vi "visuallyInspectPositionListResults2.vi"() -> ()   [LabVIEW 2016]
uses:
  <vilib>/Utility/file.llb/Write Delimited Spreadsheet (DBL).vi
  <vilib>/regexp/Match Regular Expression.xnode
  <vilib>/vision/driver/NI_Vision_Acquisition_Software.lvlib
  <vilib>/vision/NI_Vision_Development_Module.lvlib
panel:
  out "Array":dbl[][](array[numeric])=[[169.71, 122.239, 18.9126], [169.219, 25.0888, 17.9835], [73.8248, 25.6014, 13.716], [74.3048, 122.763, 15.0633], [169.71, 122.239, 18.9126], [169.219, 25.0888, 17.9835], [73.8248, 25.6014, 13.716], [74.3048, 122.763, 15.0633], [169.71, 122.239, 18.9126], [169.219, 25.0888, 17.9835], [73.8248, 25.6014, 13.716], [74.3048, 122.763, 15.0633], [169.71, 122.239, 18.9126], [169.219, 25.0888, 17.9835], [73.8248, 25.6014, 13.716], [74.3048, 122.763, 15.0633], [169.71, 122.239, 18.9126], [169.219, 25.0888, 17.9835], [73.8248, 25.6014, 13.716], [74.3048, 122.763, 15.0633], [169.71, 122.239, 18.9126], [169.219, 25.0888, 17.9835], [73.8248, 25.6014, 13.716], [74.3048, 122.763, 15.0633], [169.71, 122.239, 18.9126], [169.219, 25.0888, 17.9835], [73.8248, 25.6014, 13.716], [74.3048, 122.763, 15.0633], [169.71, 122.239, 18.9126], [169.219, 25.0888, 17.9835], [73.8248, 25.6014, 13.716], [74.3048, 122.763, 15.0633], [169.71, 122.239, 18.9126], [169.219, 25.0888, 17.9835], [73.8248, 25.6014, 13.716], [74.3048, 122.763, 15.0633], [169.71, 122.239, 18.9126], [169.219, 25.0888, 17.9835], [73.8248, 25.6014, 13.716], [74.3048, 122.763, 15.0633]]
  in  "Tab Control":T1(tab)
  in  "Path to save collected images":path=path "C:/Users/Aerotech/Downloads/Test"
  in  "List of Interesting Locations":path=path "C:/Users/Aerotech/Downloads/Test/coords.csv"
  out "Pixel Y":dbl=1374.0
  out "Pixel X":dbl=1920.0
  in  "Nloops":i32=1
  in  "Ncaptures":i32=1
  in  "File delimiter":string=","
  out "Number of Images":i32=160
  in  "Camera gain":dbl(slide)=3.6197718631178706 scale=0.0..16.0
  out "Thermometer [C]":dbl(slide)=nan scale=0.0..50.0
  in  "Coaxial light":bool
  in  "Spotlights":bool
  out "XYZ Stage Current Position":T2={"X [-750, 750 mm]"=74.30480031245196, "Y [-150, 30 mm]"=122.76299520213085, "Z [-50, 50 mm]"=15.0633357184}
  out "Finished!":bool
  in  "Home?":bool
  in  "Focusing test range [mm]":dbl=0.8
  in  "Stepsize [um]":dbl=200.0
  in  "Scan height?":bool
  in  "Axes Speeds [mm/s]":T3={"X Speed"=30.0, "Y Speed"=30.0, "Z Speed"=15.0}
  in  "Milliseconds to Wait":u32=5000
  in  "Camera Name":refnum<k21>="cam0" caption="IMAQdx Session"
  in  "Object Location [mm]":T4={"Go to X"=74.3048, "Go to Y"=122.763, "Go to Z"=15.0633}
  out "Moving":bool
  in  "Set of Coordinates to Process":dbl[][](array[numeric])=[[169.71, 122.239, 18.9126], [169.71, 122.239, 18.9126], [169.71, 122.239, 18.9126], [169.71, 122.239, 18.9126], [169.219, 25.0888, 17.9835], [169.219, 25.0888, 17.9835], [169.219, 25.0888, 17.9835], [169.219, 25.0888, 17.9835], [73.8248, 25.6014, 13.716], [73.8248, 25.6014, 13.716], [73.8248, 25.6014, 13.716], [73.8248, 25.6014, 13.716], [74.3048, 122.763, 15.0633], [74.3048, 122.763, 15.0633], [74.3048, 122.763, 15.0633], [74.3048, 122.763, 15.0633], [169.71, 122.239, 18.9126], [169.71, 122.239, 18.9126], [169.71, 122.239, 18.9126], [169.71, 122.239, 18.9126], [169.219, 25.0888, 17.9835], [169.219, 25.0888, 17.9835], [169.219, 25.0888, 17.9835], [169.219, 25.0888, 17.9835], [73.8248, 25.6014, 13.716], [73.8248, 25.6014, 13.716], [73.8248, 25.6014, 13.716], [73.8248, 25.6014, 13.716], [74.3048, 122.763, 15.0633], [74.3048, 122.763, 15.0633], [74.3048, 122.763, 15.0633], [74.3048, 122.763, 15.0633], [169.71, 122.239, 18.9126], [169.71, 122.239, 18.9126], [169.71, 122.239, 18.9126], [169.71, 122.239, 18.9126], [169.219, 25.0888, 17.9835], [169.219, 25.0888, 17.9835], [169.219, 25.0888, 17.9835], [169.219, 25.0888, 17.9835], [73.8248, 25.6014, 13.716], [73.8248, 25.6014, 13.716], [73.8248, 25.6014, 13.716], [73.8248, 25.6014, 13.716], [74.3048, 122.763, 15.0633], [74.3048, 122.763, 15.0633], [74.3048, 122.763, 15.0633], [74.3048, 122.763, 15.0633], [169.71, 122.239, 18.9126], [169.71, 122.239, 18.9126], [169.71, 122.239, 18.9126], [169.71, 122.239, 18.9126], [169.219, 25.0888, 17.9835], [169.219, 25.0888, 17.9835], [169.219, 25.0888, 17.9835], [169.219, 25.0888, 17.9835], [73.8248, 25.6014, 13.716], [73.8248, 25.6014, 13.716], [73.8248, 25.6014, 13.716], [73.8248, 25.6014, 13.716], [74.3048, 122.763, 15.0633], [74.3048, 122.763, 15.0633], [74.3048, 122.763, 15.0633], [74.3048, 122.763, 15.0633], [169.71, 122.239, 18.9126], [169.71, 122.239, 18.9126], [169.71, 122.239, 18.9126], [169.71, 122.239, 18.9126], [169.219, 25.0888, 17.9835], [169.219, 25.0888, 17.9835], [169.219, 25.0888, 17.9835], [169.219, 25.0888, 17.9835], [73.8248, 25.6014, 13.716], [73.8248, 25.6014, 13.716], [73.8248, 25.6014, 13.716], [73.8248, 25.6014, 13.716], [74.3048, 122.763, 15.0633], [74.3048, 122.763, 15.0633], [74.3048, 122.763, 15.0633], [74.3048, 122.763, 15.0633], [169.71, 122.239, 18.9126], [169.71, 122.239, 18.9126], [169.71, 122.239, 18.9126], [169.71, 122.239, 18.9126], [169.219, 25.0888, 17.9835], [169.219, 25.0888, 17.9835], [169.219, 25.0888, 17.9835], [169.219, 25.0888, 17.9835], [73.8248, 25.6014, 13.716], [73.8248, 25.6014, 13.716], [73.8248, 25.6014, 13.716], [73.8248, 25.6014, 13.716], [74.3048, 122.763, 15.0633], [74.3048, 122.763, 15.0633], [74.3048, 122.763, 15.0633], [74.3048, 122.763, 15.0633], [169.71, 122.239, 18.9126], [169.71, 122.239, 18.9126], [169.71, 122.239, 18.9126], [169.71, 122.239, 18.9126], [169.219, 25.0888, 17.9835], [169.219, 25.0888, 17.9835], [169.219, 25.0888, 17.9835], [169.219, 25.0888, 17.9835], [73.8248, 25.6014, 13.716], [73.8248, 25.6014, 13.716], [73.8248, 25.6014, 13.716], [73.8248, 25.6014, 13.716], [74.3048, 122.763, 15.0633], [74.3048, 122.763, 15.0633], [74.3048, 122.763, 15.0633], [74.3048, 122.763, 15.0633], [169.71, 122.239, 18.9126], [169.71, 122.239, 18.9126], [169.71, 122.239, 18.9126], [169.71, 122.239, 18.9126], [169.219, 25.0888, 17.9835], [169.219, 25.0888, 17.9835], [169.219, 25.0888, 17.9835], [169.219, 25.0888, 17.9835], [73.8248, 25.6014, 13.716], [73.8248, 25.6014, 13.716], [73.8248, 25.6014, 13.716], [73.8248, 25.6014, 13.716], [74.3048, 122.763, 15.0633], [74.3048, 122.763, 15.0633], [74.3048, 122.763, 15.0633], [74.3048, 122.763, 15.0633], [169.71, 122.239, 18.9126], [169.71, 122.239, 18.9126], [169.71, 122.239, 18.9126], [169.71, 122.239, 18.9126], [169.219, 25.0888, 17.9835], [169.219, 25.0888, 17.9835], [169.219, 25.0888, 17.9835], [169.219, 25.0888, 17.9835], [73.8248, 25.6014, 13.716], [73.8248, 25.6014, 13.716], [73.8248, 25.6014, 13.716], [73.8248, 25.6014, 13.716], [74.3048, 122.763, 15.0633], [74.3048, 122.763, 15.0633], [74.3048, 122.763, 15.0633], [74.3048, 122.763, 15.0633], [169.71, 122.239, 18.9126], [169.71, 122.239, 18.9126], [169.71, 122.239, 18.9126], [169.71, 122.239, 18.9126], [169.219, 25.0888, 17.9835], [169.219, 25.0888, 17.9835], [169.219, 25.0888, 17.9835], [169.219, 25.0888, 17.9835], [73.8248, 25.6014, 13.716], [73.8248, 25.6014, 13.716], [73.8248, 25.6014, 13.716], [73.8248, 25.6014, 13.716], [74.3048, 122.763, 15.0633], [74.3048, 122.763, 15.0633], [74.3048, 122.763, 15.0633], [74.3048, 122.763, 15.0633]]
  in  "Settings":T5={"Algorithm"=2, "Number of Matches Requested"=1, "Minimum Match Score"=800.0, "SubPixel Accuracy"=TRUE, "Rotation Angle Ranges"=[], "Show Search Area"=FALSE, "Show Result"=TRUE} {"Rotation Angle Ranges"."End" format="%.1f"; "Rotation Angle Ranges"."Start" format="%.1f"; "Minimum Match Score" min=0 max=1000 format="%.2f"; "Number of Matches Requested" min=1; "Algorithm" items=["All", "Low Discrepancy Sampling", "Grayscale Value Pyramid", "Gradients Pyramid"]}
  out "Most recently collected image":T6(plugin-control)
  out "Image #":i32=159
  in  "error in (no error)":errorcluster
  out "Error report":errorcluster
  out "VISA error out":errorcluster={"status"=TRUE, "code"=5002, "source"="Init.vi.  Unable to establish connection with Arduino.  Please ensure that you have selected the correct COM port and that you have flashed the Arduino with the correct firmware."}
  # "This VI can take pictures save the coordinates \nIt can also do the pattern matching at fly\nDifferent pattern could be matched but the template must be in the correct folder\nThe matched coordinates are in pixel which is to be later connverted into mm"
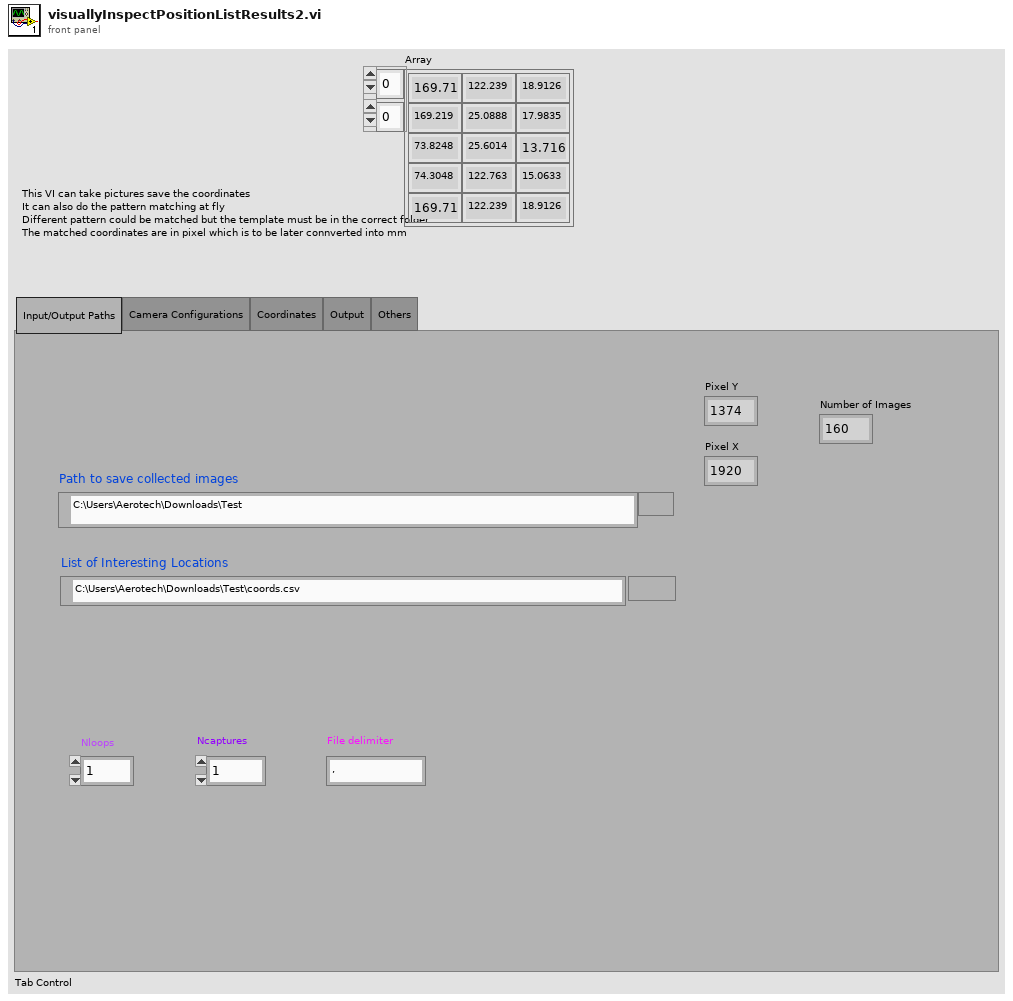
[diagram p1: front panel]
types:
  T1 = enum32{"Input/Output Paths", "Camera Configurations", "Coordinates", "Output", "Others"}
  T2 = cluster{"X [-750, 750 mm]":dbl, "Y [-150, 30 mm]":dbl, "Z [-50, 50 mm]":dbl}
  T3 = cluster{"X Speed":dbl, "Y Speed":dbl, "Z Speed":dbl}
  T4 = cluster{"Go to X":dbl, "Go to Y":dbl, "Go to Z":dbl}
  T5 = cluster{"Algorithm":i32, "Number of Matches Requested":i32, "Minimum Match Score":sgl, "SubPixel Accuracy":bool, "Rotation Angle Ranges":cluster{"Start":sgl, "End":sgl}[], "Show Search Area":bool, "Show Result":bool}
  T6 = typedef "IMAQ Image.ctl" = refnum<image>
  T7 = cluster{"Loaded array[0]":dbl, "Loaded array[1]":dbl, "Loaded array[2]":dbl, "Loaded array[3]":dbl, "Loaded array[4]":dbl, "Loaded array[5]":dbl, "Loaded array[6]":dbl, "Loaded array[7]":dbl, "Loaded array[8]":dbl}
  T8 = typedef "LabVIEW Interface for Arduino.lvlib/Arduino Resource.ctl" = cluster{"VISA resource":refnum<visa-resource-name>, "Board Type":T9, "Connection Type":enum8{"USB / Serial"}, "Bytes Per Packet (15)":u8}
  T9 = typedef "LabVIEW Interface for Arduino.lvlib/Board Type.ctl" = enum16{"Uno", "Dimuelanove w/Atmega 328", "Mega 2560"}
  T10 = typedef "ArduinoLT-ConfigurationControl.ctl" = cluster{"Lights: Digital I/O Pins":cluster{"Coaxial":u8, "Spotlights":u8}, "Thermistor Settings":cluster{"Analogue Readout Pin":u8, "Vcc Reference Pin":u8, "Paired Resistance (10K Ohms)":dbl, "Units (C)":enum16{"Celsius", "Fahrenheit", "Kelvin"}}}
  T11 = typedef "IMAQdx.ctl" = refnum<k21>
  T12 = cluster{"Set of Coordinates to Process[0]":dbl, "Set of Coordinates to Process[1]":dbl, "Set of Coordinates to Process[2]":dbl}
  T13 = typedef "Image Type" = u32
  T14 = cluster{"Final X":dbl, "Final Y":dbl, "Final Z":dbl}
  T15 = cluster{"Position":cluster{"x":sgl, "y":sgl}, "Angle":sgl, "Scale":sgl, "Score":sgl, "Bounding Box":cluster{"x":sgl, "y":sgl}[]}[]
  T16 = cluster{"Matches (pixel)[0]":cluster{"Position":cluster{"x":sgl, "y":sgl}, "Angle":sgl, "Scale":sgl, "Score":sgl, "Bounding Box":cluster{"x":sgl, "y":sgl}[]}, "Matches (pixel)[1]":cluster{"Position":cluster{"x":sgl, "y":sgl}, "Angle":sgl, "Scale":sgl, "Score":sgl, "Bounding Box":cluster{"x":sgl, "y":sgl}[]}, "Matches (pixel)[2]":cluster{"Position":cluster{"x":sgl, "y":sgl}, "Angle":sgl, "Scale":sgl, "Score":sgl, "Bounding Box":cluster{"x":sgl, "y":sgl}[]}, "Matches (pixel)[3]":cluster{"Position":cluster{"x":sgl, "y":sgl}, "Angle":sgl, "Scale":sgl, "Score":sgl, "Bounding Box":cluster{"x":sgl, "y":sgl}[]}, "Matches (pixel)[4]":cluster{"Position":cluster{"x":sgl, "y":sgl}, "Angle":sgl, "Scale":sgl, "Score":sgl, "Bounding Box":cluster{"x":sgl, "y":sgl}[]}, "Matches (pixel)[5]":cluster{"Position":cluster{"x":sgl, "y":sgl}, "Angle":sgl, "Scale":sgl, "Score":sgl, "Bounding Box":cluster{"x":sgl, "y":sgl}[]}, "Matches (pixel)[6]":cluster{"Position":cluster{"x":sgl, "y":sgl}, "Angle":sgl, "Scale":sgl, "Score":sgl, "Bounding Box":cluster{"x":sgl, "y":sgl}[]}, "Matches (pixel)[7]":cluster{"Position":cluster{"x":sgl, "y":sgl}, "Angle":sgl, "Scale":sgl, "Score":sgl, "Bounding Box":cluster{"x":sgl, "y":sgl}[]}, "Matches (pixel)[8]":cluster{"Position":cluster{"x":sgl, "y":sgl}, "Angle":sgl, "Scale":sgl, "Score":sgl, "Bounding Box":cluster{"x":sgl, "y":sgl}[]}}
  T17 = cluster{"Position":cluster{"x":sgl, "y":sgl}, "Angle":sgl, "Scale":sgl, "Score":sgl, "Bounding Box":cluster{"x":sgl, "y":sgl}[]}
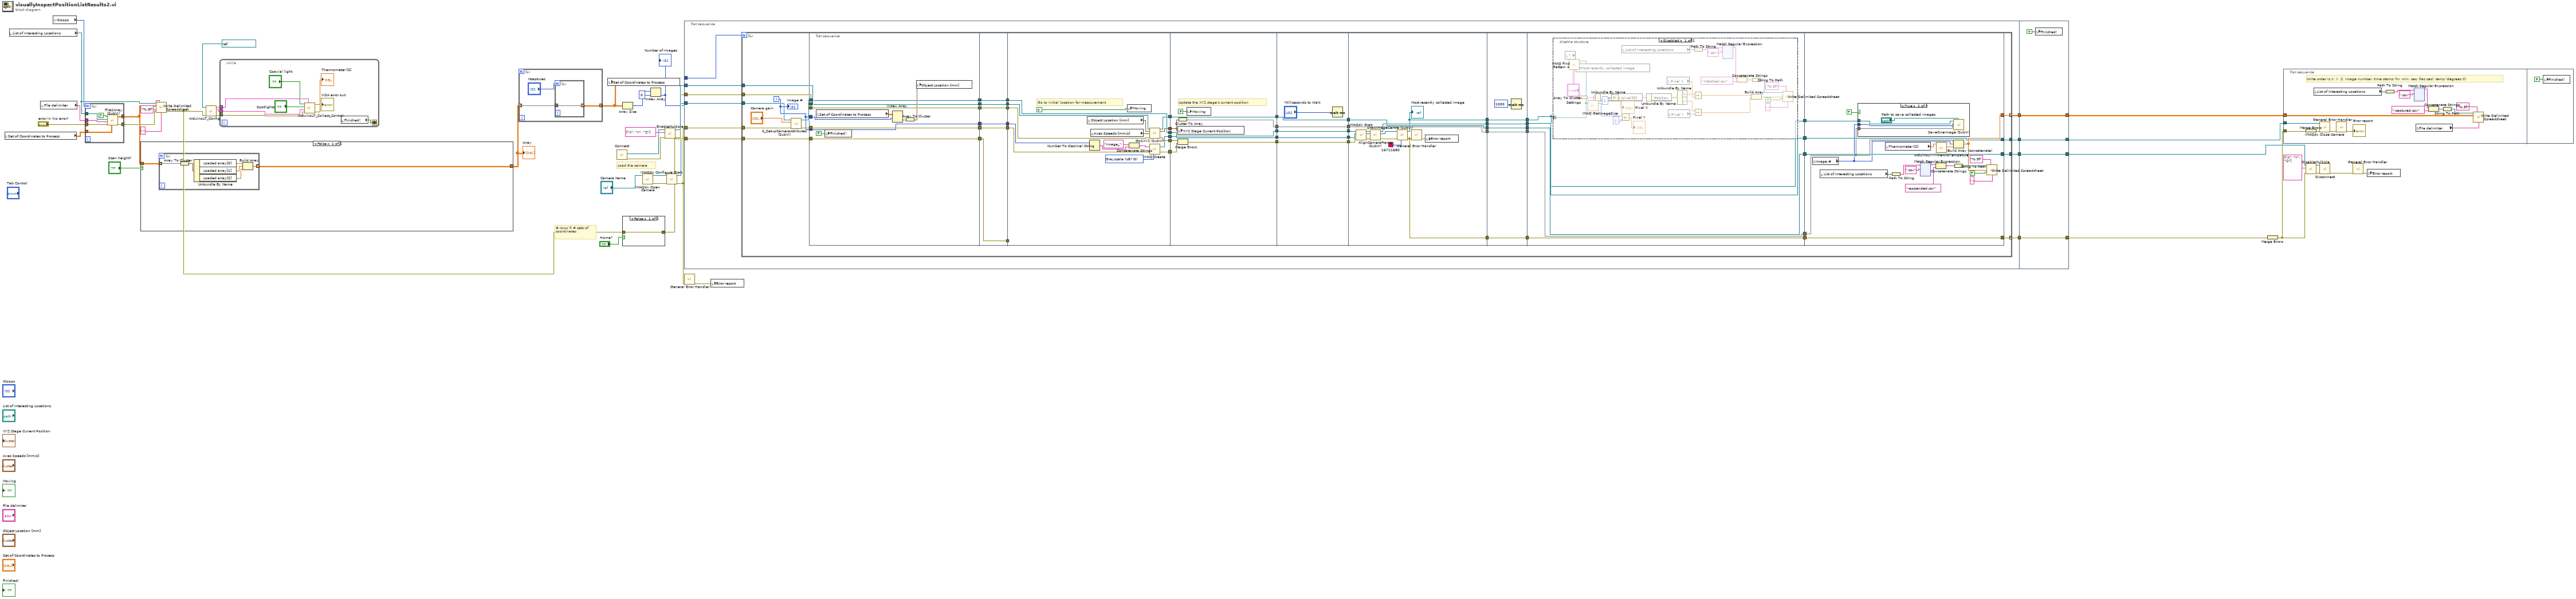
[diagram p0: block diagram]
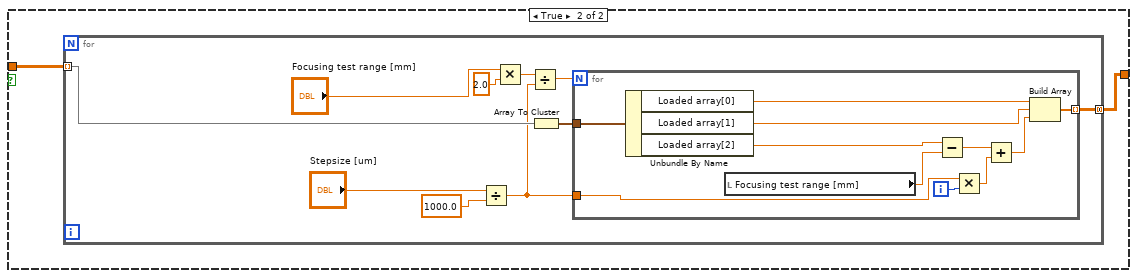
[diagram p2: hidden frame]
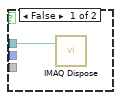
[diagram p4: hidden frame]
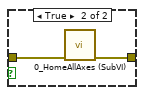
[diagram p5: hidden frame]
diagram:
  # "# rows = # sets of\ncoordinates"
  # "Load the camera"
  n1 = local read "Set of Coordinates to Process"() -> (w36:dbl[][])
  n2 = local read "List of Interesting Locations"() -> (w35:path)
  n3 = local read "File delimiter"() -> (w38:string)
  n4 = local read "Nloops"() -> (w15:i32)
  n5 = for {
    N: w15 -> [_]
    tunnel: w35 -> [w51]
    tunnel: w38 -> [w50]
    tunnel: w36 -> [w48]
    tunnel: [w54] -> w17 mode=concatenating
    tunnel: "error in (no error)" -> [w49]
    tunnel: [w53] -> w13
    n6 = call "File2Array (SubVI).vi"("Array for Processing"=w48, "error in (no error) in"=w49, "File delimiter"=w50, "Source array file"=w51, "Load array from file?"=TRUE) -> ("error in (no error) out"=w53:errorcluster, "Loaded array"=w54:dbl[][])  [unwired: 5 in]
  }
  n7 = case shown="False" "Scan height?" {
    tunnel: w17 -> [w56 w64]
    tunnel: [w55 w63] -> w16
    frame False {
      n8 = for {
        tunnel: w56 -> [w62] mode=indexing
        tunnel: [w58] -> w55 mode=indexing
        n9 = Array To Cluster(array=w62) -> (cluster=w61:T7)
        n10 = Unbundle By Name(w61) -> ("Loaded array[0]"=w60:dbl, "Loaded array[1]"=w59:dbl, "Loaded array[2]"=w57:dbl)
        n11 = Build Array(w60, w59, w57) -> (w58:dbl[])
      }
    }
    frame True {
      n12 = for {
        tunnel: w64 -> [w70] mode=indexing
        tunnel: [w68] -> w63 mode=concatenating
        n13 = Divide(x="Stepsize [um]", y=1000.0) -> (x/y=w65:dbl)
        n14 = Multiply(x="Focusing test range [mm]", y=2.0) -> (x*y=w72:dbl)
        n15 = Divide(x=w72, y=w65) -> (x/y=w73:dbl)
        n16 = Array To Cluster(array=w70) -> (cluster=w69:T7)
        n17 = for {
          N: w73 -> [_]
          tunnel: w69 -> [w85]
          tunnel: [w82] -> w68 mode=indexing
          tunnel: w65 -> [w80]
          i -> [w81]
          n18 = Unbundle By Name(w85) -> ("Loaded array[0]"=w84:dbl, "Loaded array[1]"=w83:dbl, "Loaded array[2]"=w79:dbl)
          n19 = local read "Focusing test range [mm]"() -> (w78:dbl)
          n20 = Subtract(x=w79, y=w78) -> (x-y=w77:dbl)
          n21 = Multiply(x=w80, y=w81) -> (x*y=w76:dbl)
          n22 = Add(x=w77, y=w76) -> (x+y=w75:dbl)
          n23 = Build Array(w84, w83, w75) -> (w82:dbl[])
        }
      }
    }
  }
  "Array" <- w16
  n24 = call-poly <vilib>:"Write Delimited Spreadsheet.vi"("file path (dialog if empty)"=w35, "format (%.3f)"="%.9f", "2D data"=w17, "error in (no error)"=w13, "delimiter (\\t)"="," ("delimiter (\\t)")) -> ("error out"=w9:errorcluster)  [unwired: 9 in, 1 out]
  n25 = call "ArduinoLT_Config.vi"("error in"=w9, "VISA resource"=refnum<visa-resource-name> "LightsCTRL") -> ("error out"=w5:errorcluster, "Arduino Resource"=w8:T8, "Arduino Configuration OUT"=w7:T10)  [unwired: 3 in, 1 out]
  n26 = while {
    tunnel: w8 -> [w89]
    tunnel: w7 -> [w88]
    tunnel: w5 -> [w87]
    stop <- w90 stop-if-true
    n27 = call "ArduinoLT_Collect_Control.vi"("Arduino Configuration"=w88, "error in"=w87, "Arduino Resource IN"=w89, "Spotlights"="Spotlights", "Coaxial light"="Coaxial light") -> ("error out"=→"VISA error out":errorcluster, "Thermometer [C]"=→"Thermometer [C]":dbl)  [unwired: 4 in, 1 out]
    n28 = local read "Finished!"() -> (w90:bool)
  }
  n29 = for {
    tunnel: w16 -> [w95] mode=indexing
    tunnel: [w94] -> w1 mode=concatenating
    n30 = for {
      N: "Ncaptures" -> [_]
      tunnel: w95 -> [w97]
      tunnel: [w97] -> w94 mode=indexing
    }
  }
  n31 = local write "Set of Coordinates to Process"(w1) -> ()
  n32 = call "Connect.vi"() -> ("error out"=w29:errorcluster, "controller"=w28:refnum<k24>)  [unwired: 10 in]
  n33 = Array Size(array=w1) -> (size(s)=w3:i32[])
  n34 = case shown="False" "Home?" {
    tunnel: w9 -> [w98 w100]
    tunnel: [w98 w99] -> w42
    frame False {
    }
    frame True {
      n35 = call "0_HomeAllAxes (SubVI).vi"("error in (no error)"=w100) -> ("error out"=w99:errorcluster)  [unwired: 7 in, 3 out]
    }
  }
  n36 = call <vilib>:"IMAQdx Open Camera.vi"("Session In"="Camera Name") -> ("error out"=w46:errorcluster, "Session Out"=w47:T11)  [unwired: 2 in, 7 out]
  n37 = Index Array(array=w3, index=0) -> (element=w2:i32)
  "Number of Images" <- w2
  n38 = call "EnableMultiple.vi"("error in (no error)"=w29, "axis names"=string[] ["X", "Y", "Z"], "controller in"=w28) -> ("error out"=w26:errorcluster, "controller out"=w27:refnum<k24>)  [unwired: 7 in]
  n39 = call <vilib>:"IMAQdx Configure Grab.vi"("error in"=w46, "Session In"=w47) -> ("error out"=w10:errorcluster, "Session Out"=w11:T11)  [unwired: 8 out]
  n40 = flat-sequence {
    tunnel: [w109] -> w34
    tunnel: [w103] -> w33
    tunnel: [w107] -> w32
    tunnel: [w104] -> w25
    tunnel: w2 -> [w110]
    tunnel: w42 -> [w108]
    tunnel: w27 -> [w106]
    tunnel: w26 -> [w105]
    tunnel: w11 -> [w102]
    tunnel: w10 -> [w101]
    tunnel: [w528] -> w41
    tunnel: [w529] -> w43
    tunnel: [w530] -> w44
    tunnel: w34 -> [w530]
    tunnel: w33 -> [w529]
    tunnel: w32 -> [w528]
    tunnel: [w526] -> w23
    tunnel: w25 -> [w526]
    frame #0 {
      n41 = for {
        N: w110 -> [_]
        tunnel: w108 -> [w157]
        tunnel: [w153] -> w109
        tunnel: [w152] -> w107 mode=indexing
        tunnel: w106 -> [w145]
        tunnel: w105 -> [w144]
        tunnel: [w140] -> w104
        tunnel: [w139] -> w103 mode=indexing
        tunnel: w102 -> [w125]
        tunnel: w101 -> [w124]
        i -> [w126]
        n42 = call "0_SetupCameraAttributes (SubVI).vi"("error in (no error)"=w124, "Gain"="Camera gain", "Camera session in"=w125) -> ("error out"=w121:errorcluster, "Camera session out"=w123:T11)  [unwired: 7 in]
        n43 = flat-sequence {
          tunnel: w126 -> [w174]
          tunnel: w126 -> [w173]
          tunnel: [w173] -> w138
          tunnel: [w172] -> w136
          tunnel: w123 -> [w172]
          tunnel: [w171] -> w134
          tunnel: w157 -> [w171]
          tunnel: [w167] -> w132
          tunnel: w121 -> [w167]
          tunnel: [w169] -> w130
          tunnel: w145 -> [w169]
          tunnel: w144 -> [w168]
          tunnel: [w168] -> w128
          tunnel: w138 -> [w183]
          tunnel: [w183] -> w137
          tunnel: w136 -> [w182]
          tunnel: [w182] -> w135
          tunnel: w134 -> [w181]
          tunnel: [w181] -> w133
          tunnel: w132 -> [w180]
          tunnel: [w180] -> w131
          tunnel: w130 -> [w179]
          tunnel: [w179] -> w129
          tunnel: w128 -> [w178]
          tunnel: [w178] -> w127
          tunnel: [w196] -> w166
          tunnel: [w195] -> w165
          tunnel: [w194] -> w164
          tunnel: w137 -> [w189]
          tunnel: [w191] -> w161
          tunnel: [w190] -> w158
          tunnel: w135 -> [w190]
          tunnel: w133 -> [_]
          tunnel: w131 -> [w187]
          tunnel: [w186] -> w154
          tunnel: w129 -> [w185]
          tunnel: w127 -> [w184]
          tunnel: w166 -> [w201]
          tunnel: w165 -> [w204]
          tunnel: w164 -> [w202]
          tunnel: [w208] -> w162
          tunnel: w161 -> [w208]
          tunnel: [w207] -> w159
          tunnel: w158 -> [w207]
          tunnel: [w205] -> w155
          tunnel: w154 -> [w206]
          tunnel: [w203] -> w151
          tunnel: [w201] -> w143
          tunnel: [w214] -> w163
          tunnel: w162 -> [w214]
          tunnel: [w213] -> w160
          tunnel: w159 -> [w213]
          tunnel: [w212] -> w156
          tunnel: w155 -> [w212]
          tunnel: w151 -> [w211]
          tunnel: [w211] -> w150
          tunnel: w143 -> [w210]
          tunnel: [w210] -> w142
          tunnel: w163 -> [w230]
          tunnel: w160 -> [w229]
          tunnel: w156 -> [w227]
          tunnel: w150 -> [w225]
          tunnel: [w220] -> w149
          tunnel: [w219] -> w148
          tunnel: [w225] -> w147
          tunnel: [w218] -> w146
          tunnel: w142 -> [w216]
          tunnel: [w216] -> w141
          tunnel: w149 -> [w236]
          tunnel: w148 -> [w235]
          tunnel: w147 -> [w234]
          tunnel: [w236] -> w115
          tunnel: [w235] -> w114
          tunnel: [w234] -> w113
          tunnel: w146 -> [w232]
          tunnel: [w232] -> w112
          tunnel: [w231] -> w111
          tunnel: w141 -> [w231]
          tunnel: w115 -> [w241]
          tunnel: [w241] -> w120
          tunnel: w114 -> [w240]
          tunnel: [w240] -> w119
          tunnel: w113 -> [w239]
          tunnel: [w239] -> w118
          tunnel: w112 -> [w237]
          tunnel: [w237] -> w117
          tunnel: w111 -> [w238]
          tunnel: [w238] -> w116
          tunnel: [w405] -> w152
          tunnel: [w406] -> w153
          tunnel: w120 -> [w406]
          tunnel: w119 -> [w405]
          tunnel: w118 -> [w402]
          tunnel: w117 -> [w404]
          tunnel: [w403] -> w140
          tunnel: w116 -> [w403]
          tunnel: [w392] -> w139
          frame #0 {
            n44 = local read "Set of Coordinates to Process"() -> (w175:dbl[][])
            n45 = local write "Finished!"(FALSE ("Finished!")) -> ()
            n46 = Index Array(array=w175, index (row)=w174) -> (element=w176:dbl[])  [unwired: 1 in]
            n47 = Array To Cluster(array=w176) -> (cluster=w177:T12)
            n48 = local write "Object Location [mm]"(w177) -> ()
          }
          frame #1 {
          }
          frame #2 {
            w200 = T13 0 items=["Grayscale (U8)", "Grayscale (I16)", "Grayscale (SGL)", "Complex (CSG)", "RGB (U32)", "HSL (U32)", "RGB (U64)", "Grayscale (U16)"] ("Image Type")
            # "Go to initial location for measurement"
            n49 = local read "Object Location [mm]"() -> (w197:T4)
            n50 = Number To Decimal String(number=w189) -> (decimal integer string=w188:string)  [unwired: 1 in]
            n51 = local read "Axes Speeds [mm/s]"() -> (w198:T3)
            n52 = local write "Moving"(TRUE ("Moving")) -> ()
            n53 = Concatenate Strings("image_" ("Image Name"), w188) -> (w192:string)
            n54 = call "Go2XYZ (SubVI).vi"(".NET Refnum in"=w185, "Go to Coordinates"=w197, "Axis Speeds"=w198, "error in (no error)"=w184) -> (".NET Refnum out"=w196:refnum<k24>, "Final Position"=w195:T14, "error out"=w194:errorcluster)  [unwired: 7 in, 2 out]
            n55 = call "IMAQ Create"("Image Name"=w192, "Image Type"=w200, "error in (no error)"=w187) -> ("New Image"=w191:T6, "error out"=w186:errorcluster)  [unwired: 1 in, 1 out]
          }
          frame #3 {
            # "Update the XYZ stage's current position"
            n56 = Cluster To Array(cluster=w204) -> (array=w203:dbl[])
            n57 = local write "XYZ Stage Current Position"(w204) -> ()
            n58 = Merge Errors(w202, w206) -> (w205:errorcluster)
            n59 = local write "Moving"(FALSE ("Moving")) -> ()
          }
          frame #4 {
            n60 = Wait (ms)(milliseconds to wait="Milliseconds to Wait") -> ()  [unwired: 1 out]
          }
          frame #5 {
            n61 = call <vilib>:"IMAQdx Grab.vi"("error in"=w227, "Image In"=w230, "Session In"=w229) -> ("error out"=w226:errorcluster, "Image Out"=w228:T6, "Session Out"=w221:T11)  [unwired: 1 in, 5 out]
            n62 = call "AlignCameraFrame (SubVI).vi"("error in (no error)"=w226, "Image Src"=w228, "Camera session in"=w221) -> ("error out"=w223:errorcluster, "Image Dst Out"=w224:T6, "Camera session out"=w220:T11)  [unwired: 6 in]
            n63 = call "DrawImageCentre (SubVI).vi"("Axis colour"=u32 16711680, "error in (no error)"=w223, "Refnum in"=w224) -> ("error out"=w219:errorcluster, "Refnum out"=w218:T6)  [unwired: 7 in]
            "Most recently collected image" <- w218
            n64 = call <vilib>:"General Error Handler.vi"("error in (no error)"=w219) -> ("error out"=w217:errorcluster)  [unwired: 2 in, 12 out]
            n65 = local write "Error report"(w217) -> ()
          }
          frame #6 {
            n66 = Wait (ms)(milliseconds to wait=u32 1000) -> ()  [unwired: 1 out]
          }
          frame #7 {
            n67 = disable-structure shown="Disabled" {
              disable-tunnel: w237 -> [w269 _]
              frame Disabled {
                n68 = local read item#-1() -> (w245)
                n69 = call "IMAQ Find Pattern 4"("Image"=w269, "Template"=w245, "Settings"="Settings") -> ("Image Out"=w268:T6, "Matches (pixel)"=w267:T15)  [unwired: 6 in, 5 out]
                n70 = local write "Most recently collected image"(w268) -> ()
                n71 = Array To Cluster(array=w267) -> (cluster=w266:T16)
                n72 = call "IMAQ GetImageSize"("Image"=w269) -> ("Y Resolution"=w242:i32, "X Resolution"=w272:i32)  [unwired: 3 in, 1 out]
                n73 = Unbundle By Name(w266) -> ("Matches (pixel)[0]"=w265:T17)
                n74 = Divide(x=w272, y=2) -> (x/y=→"Pixel X":dbl)
                n75 = Divide(x=w242, y=2) -> (x/y=→"Pixel Y":dbl)
                n76 = local read "List of Interesting Locations"() -> (w251:path)
                n77 = Unbundle By Name(w265) -> ("Position"=w264:cluster{"x":sgl, "y":sgl})
                n78 = local read "Pixel X"() -> (w262:dbl)
                n79 = local read "Pixel Y"() -> (w260:dbl)
                n80 = Unbundle By Name(w264) -> ("x"=w263:sgl, "y"=w261:sgl)
                n81 = Subtract(x=w263, y=w262) -> (x-y=w259:dbl)
                n82 = Subtract(x=w261, y=w260) -> (x-y=w258:dbl)
                n83 = Path To String(path=w251) -> (string=w252:string)
                n84 = xnode "Match Regular Expression"("input string"=w252, "regular expression"=".csv") -> ("before match"=w255:string)  [unwired: 4 in, 4 out]
                n85 = Concatenate Strings(w255, "-Matched.csv" ("name or relative path")) -> (w256:string)
                n86 = String To Path(string=w256) -> (path=w257:path)
                n87 = Build Array(w259, w258) -> (w248:dbl[])
                n88 = call-poly <vilib>:"Write Delimited Spreadsheet.vi"("file path (dialog if empty)"=w257, "format (%.3f)"="%.9f", "1D data"=w248, "append to file? (new file:F)"=TRUE, "delimiter (\\t)"="," ("delimiter (\\t)")) -> ()  [unwired: 9 in, 2 out]
              }
              frame Enabled {
              }
            }
          }
          frame #8 {
            n89 = local read "Image #"() -> (w401:i32)
            n90 = local read "List of Interesting Locations"() -> (w400:path)
            n91 = case shown="True" TRUE {
              tunnel: w404 -> [w407 w411]
              tunnel: w402 -> [_ w409]
              tunnel: w401 -> [_ w408]
              frame False {
                n92 = call "IMAQ Dispose"("Image"=w407) -> ()  [unwired: 5 in, 1 out]
              }
              frame True {
                n93 = call "SaveOneImage (SubVI).vi"("Save images path"="Path to save collected images", "XYZ stage coordinates of image"=w409, "Image Number"=w408, "Image"=w411) -> ()  [unwired: 7 in, 1 out]
              }
            }
            n94 = local read "Thermometer [C]"() -> (w388:dbl)
            n95 = Path To String(path=w400) -> (string=w399:string)
            n96 = xnode "Match Regular Expression"("input string"=w399, "regular expression"=".csv") -> ("before match"=w396:string)  [unwired: 4 in, 4 out]
            n97 = Concatenate Strings(w396, "-appended.csv" ("name or relative path")) -> (w395:string)
            n98 = call "ArduinoLT-TimeAndTempature.vi"("Temperature"=w388) -> ("double( Time, Temp )"=w389:dbl[])  [unwired: 8 in, 2 out]
            n99 = String To Path(string=w395) -> (path=w394:path)
            n100 = Build Array (concatenate)(w402, w401, w389) -> (w392:dbl[])
            n101 = call-poly <vilib>:"Write Delimited Spreadsheet.vi"("file path (dialog if empty)"=w394, "format (%.3f)"="%.9f", "1D data"=w392, "append to file? (new file:F)"=TRUE, "delimiter (\\t)"="," ("delimiter (\\t)")) -> ()  [unwired: 9 in, 2 out]
          }
        }
        "Image #" <- w126
      }
    }
    frame #1 {
      n102 = local write "Finished!"(TRUE ("Finished!")) -> ()
    }
  }
  n103 = call <vilib>:"General Error Handler.vi"("error in (no error)"=w10) -> ("error out"=w40:errorcluster)  [unwired: 2 in, 12 out]
  n104 = local write "Error report"(w40) -> ()
  n105 = Merge Errors(w41) -> (w21:errorcluster)
  n106 = flat-sequence {
    tunnel: w21 -> [w535]
    tunnel: w44 -> [w534]
    tunnel: w43 -> [w533]
    frame #0 {
      # "Write order is X, Y, Z, image number, time stamp (hr, min, sec, frac sec), temp (degrees C)"
      n107 = Merge Errors(w535) -> (w536:errorcluster)
      n108 = local read "List of Interesting Locations"() -> (w538:path)
      n109 = call <vilib>:"IMAQdx Close Camera.vi"("error in"=w536, "Session In"=w534) -> ("error out"=w532:errorcluster)  [unwired: 9 out]
      n110 = call <vilib>:"General Error Handler.vi"("error in (no error)"=w532) -> ("error out"=→"Error report":errorcluster)  [unwired: 2 in, 12 out]
      n111 = Path To String(path=w538) -> (string=w539:string)
      n112 = xnode "Match Regular Expression"("input string"=w539, "regular expression"=".csv") -> ("before match"=w542:string)  [unwired: 4 in, 4 out]
      n113 = local read "File delimiter"() -> (w545:string)
      n114 = Concatenate Strings(w542, "-captured.csv" ("name or relative path")) -> (w543:string)
      n115 = String To Path(string=w543) -> (path=w544:path)
      n116 = call-poly <vilib>:"Write Delimited Spreadsheet.vi"("file path (dialog if empty)"=w544, "format (%.3f)"="%.9f", "2D data"=w533, "delimiter (\\t)"=w545) -> ()  [unwired: 10 in, 2 out]
    }
    frame #1 {
      n117 = local write "Finished!"(FALSE ("Finished!")) -> ()
    }
  }
  n118 = call "DisableMultiple.vi"("error in (no error)"=w21, "axis names"=string[] ["X", "Y", "Z"], "controller in"=w23) -> ("error out"=w20:errorcluster, "controller out"=w22:refnum<k24>)  [unwired: 7 in]
  n119 = call "Disconnect.vi"("error in (no error)"=w20, "controller"=w22) -> ("error out"=w24:errorcluster)  [unwired: 9 in]
  n120 = call <vilib>:"General Error Handler.vi"("error in (no error)"=w24) -> ("error out"=w31:errorcluster)  [unwired: 2 in, 12 out]
  n121 = local write "Error report"(w31) -> ()
